vi "Set Enable Rmb User.vi"(8 "error in (no error)":errorcluster, 10 "enable rmb user":bool, 11 "[Data] Recent User in":refnum<class "[Data] Recent User.lvclass">) -> (0 "error out":errorcluster, 3 "[Data] Recent User out":refnum<class "[Data] Recent User.lvclass">)   [LabVIEW 2020, in "[Data] Recent User.lvclass"]
uses:
  [Data] Recent User.lvclass
  [Data] Recent User.lvclass/[Data] Recent User.ctl
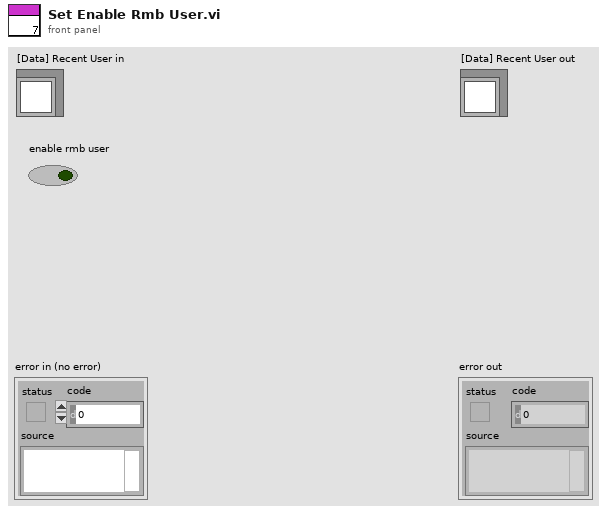
[diagram p1: front panel]
types:
  T1 = cluster{"enable rmb user":bool, "recent user list":string[]}
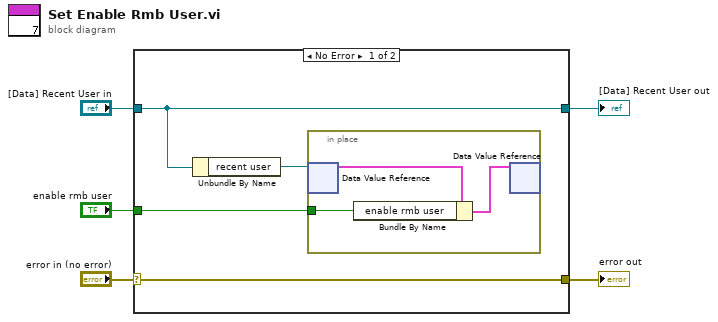
[diagram p0: block diagram]
diagram:
  n1 = case shown="No Error" "error in (no error)" {
    selector: "error in (no error)" -> [w9 w14]
    tunnel: [w9 w14] -> w4
    tunnel: [w8 w13] -> w2
    tunnel: "[Data] Recent User in" -> [w8 w13]
    tunnel: "enable rmb user" -> [w6 _]
    frame No Error {
      n2 = Unbundle By Name(w8) -> ("recent user"=w7:refnum<data-value>)
      n3 = in-place {
        in-place-border: w6 -> [w11]
        n4 = in-place-dvr #1(w7) -> (w12:T1)  [unwired: 1 out]
        n5 = Bundle By Name(cluster=w12, "enable rmb user"=w11) -> (w10:T1)
        n6 = in-place-dvr #1(w10) -> ()  [unwired: 2 out]
      }
    }
    frame Error {
    }
  }
  "error out" <- w4
  "[Data] Recent User out" <- w2
